vi "Messages.vi"() -> (3 ";)   ?":dbl caption="С колко?" format="%#g")   [LabVIEW 2023]
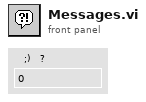
[diagram p1: front panel]
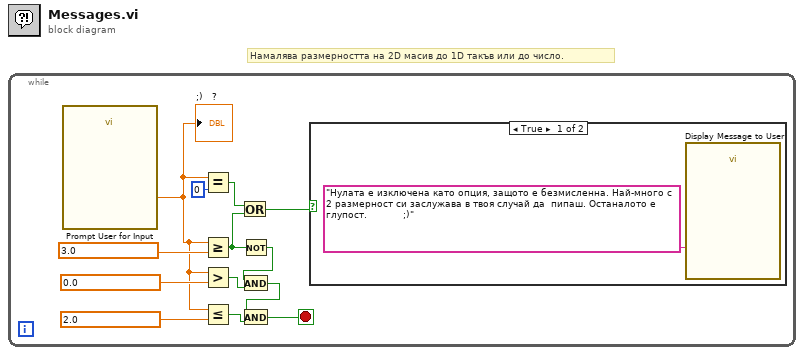
[diagram p0: block diagram]
diagram:
  # "Намалява размерността на 2D масив до 1D такъв или до число."
  n1 = while {
    stop <- w6 stop-if-true
    n2 = call "Prompt User for Input"() -> ("Препоръчително е да избереш максимум 2!"=w5:dbl)  [unwired: 17 in, 2 out]
    ";)   ?" <- w5
    n3 = Equal?(x=w5, y=u64 0) -> (x = y?=w3:bool)
    n4 = Greater Or Equal?(x=w5, y=3.0) -> (x >= y?=w2:bool)
    n5 = Greater?(x=w5, y=0.0) -> (0:w9:bool)
    n6 = Less Or Equal?(x=w5, y=2.0) -> (x <= y?=w7:bool)
    n7 = Or(x=w3, y=w2) -> (x .or. y?=w1:bool)
    n8 = Not(x=w2) -> (.not. x?=w10:bool)
    n9 = And(x=w10, y=w9) -> (x .and. y?=w8:bool)
    n10 = And(x=w8, y=w7) -> (x .and. y?=w6:bool)
    n11 = case shown="True" w1 {
      frame True {
        n12 = call "Display Message to User"("Message"="Нулата е изключена като опция, защото е безмисленна. Най-много с 2 размерност си заслужава в твоя случай да  пипаш. Останалото е глупост.            ;)") -> ()  [unwired: 9 in, 2 out]
      }
      frame False {
      }
    }
  }
